vi "Check Tlg.vi"(0 "Data Read In":T1[](array[typedef]) {"FlexRay"."cycle count" max=63 step=1; "payload" format="%x"; "identifier / slot" format="%x"}, 7 "Tlg Data Array":T2 {"CAN frame In"."FlexRay"."cycle count" max=63 step=1; "CAN frame In"."payload" format="%x"; "CAN frame In"."identifier / slot" format="%x"; "FlexRay Channel" items=["A", "B", "A+B"]}, 11 "Error In":errorcluster {"code" format="%.0x"}) -> (4 "Data Read Out":T1[](array[typedef]) {"FlexRay"."cycle count" max=63 step=1; "payload" format="%x"; "identifier / slot" format="%x"}, 8 "Tlg Data Array out":T2 {"CAN frame In"."FlexRay"."cycle count" max=63 step=1; "CAN frame In"."payload" format="%x"; "CAN frame In"."identifier / slot" format="%x"; "FlexRay Channel" items=["A", "B", "A+B"]}, 15 "Error out":errorcluster {"code" format="%.0x"})   [LabVIEW 2014, in "CAN Bus Monitor Engine.lvlib"]
uses:
  CAN Bus Monitor Engine.lvlib
  Controls/Analyze Array.ctl
  Controls/FlexRay Channel.ctl
  Controls/XNET BM Frame.ctl
panel:
  in  "ActualEntry":u32
  in  "EntryFound":bool
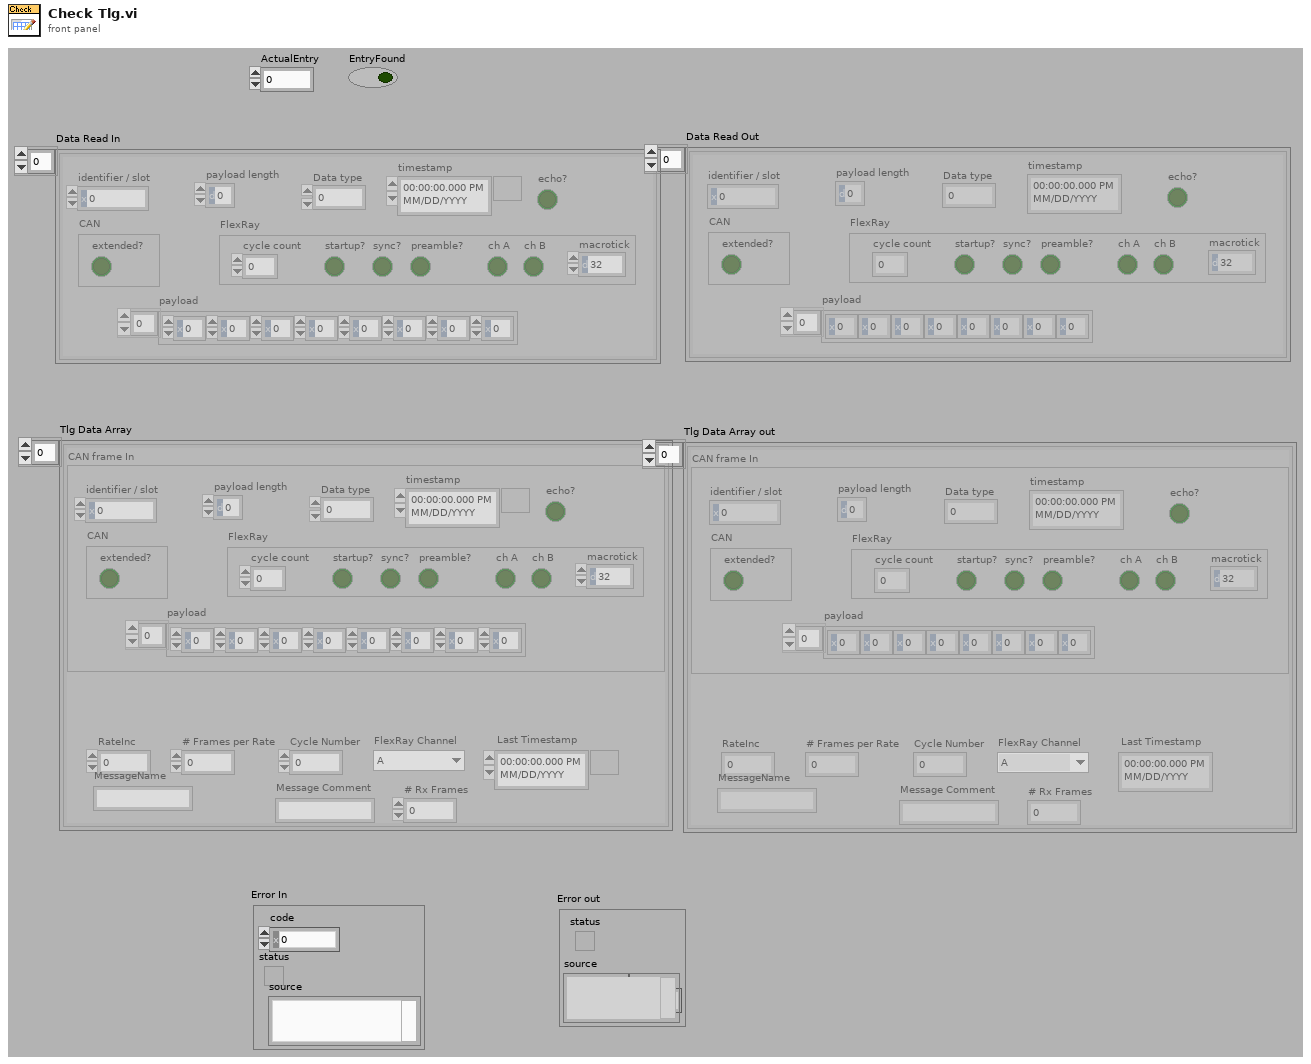
[diagram p1: front panel]
types:
  T1 = typedef "CAN Bus Monitor Engine.lvlib/XNET BM Frame.ctl" = cluster{"timestamp":timestamp, "payload":u8[], "identifier / slot":u32, "Data type":u8, "payload length":u8, "CAN":cluster{"extended?":bool}, "FlexRay":cluster{"cycle count":u8, "startup?":bool, "sync?":bool, "preamble?":bool, "ch A":bool, "ch B":bool, "macrotick":u16}, "echo?":bool}
  T2 = typedef "CAN Bus Monitor Engine.lvlib/Analyze Array.ctl" = cluster{"# Rx Frames":u32, "Last Timestamp":timestamp, "RateInc":dbl, "# Frames per Rate":u32, "MessageName":string, "Cycle Number":u32, "FlexRay Channel":T3, "Message Comment":string, "CAN frame In":T1}[]
  T3 = typedef "CAN Bus Monitor Engine.lvlib/FlexRay Channel.ctl" = u16
  T4 = cluster{"# Rx Frames":u32, "Last Timestamp":timestamp, "RateInc":dbl, "# Frames per Rate":u32, "MessageName":string, "Cycle Number":u32, "FlexRay Channel":T3, "Message Comment":string, "CAN frame In":T1}
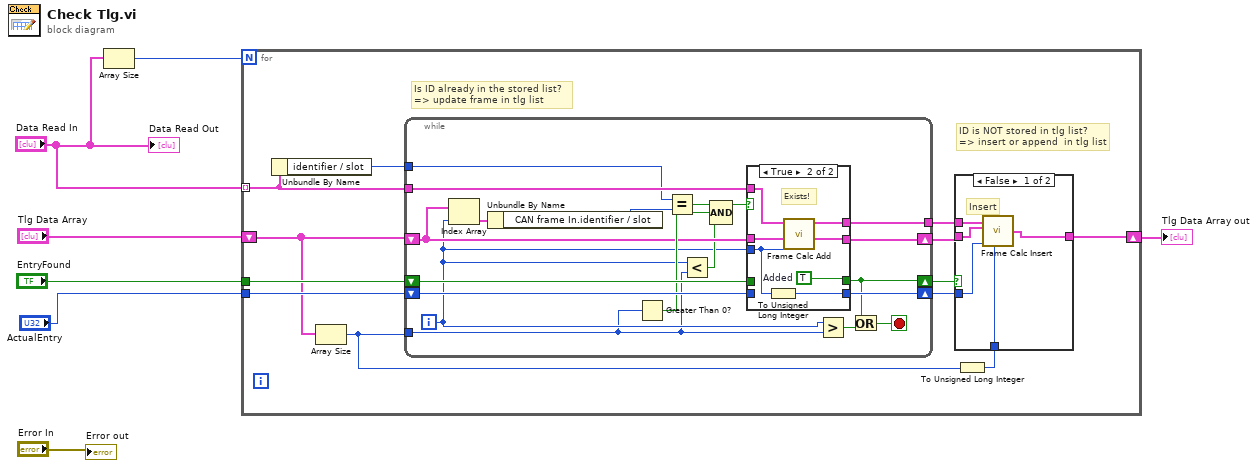
[diagram p0: block diagram]
diagram:
  n1 = Array Size(array="Data Read In") -> (size(s)=w1:i32)
  n2 = for {
    N: w1 -> [_]
    tunnel: "EntryFound" -> [w19]
    tunnel: "Data Read In" -> [w9] mode=indexing
    tunnel: "ActualEntry" -> [w17]
    shift-right: [w18] -> w4
    shift-left: "Tlg Data Array" -> [w11]
    # "ID is NOT stored in tlg list?\n=> insert or append  in tlg list"
    # "Is ID already in the stored list?\n=> update frame in tlg list"
    n3 = Unbundle By Name(w9) -> ("identifier / slot"=w12:u32)
    n4 = Array Size(array=w11) -> (size(s)=w10:i32)
    n5 = while {
      tunnel: w9 -> [w35]
      shift-right: [w40] -> w15
      shift-left: w17 -> [w41]
      shift-right: [w36] -> w14
      shift-left: w19 -> [w44]
      tunnel: w10 -> [w26]
      tunnel: [w34] -> w13
      shift-right: [w39] -> w16
      shift-left: w11 -> [w30]
      tunnel: w12 -> [w31]
      i -> [w27]
      stop <- w38 stop-if-true
      n6 = Index Array(array=w30, index=w27) -> (element=w29:T4)
      n7 = Unbundle By Name(w29) -> ("CAN frame In.identifier / slot"=w42:u32)
      n8 = Greater Than 0?(x=w26) -> (x > 0?=w32:bool)
      n9 = Equal?(x=w31, y=w42) -> (x = y?=w43:bool)
      n10 = Less?(x=w27, y=w26) -> (x < y?=w28:bool)
      n11 = Compound Arithmetic op=AND(w43, w32, w28) -> (w33:bool)
      n12 = case shown="True" w33 {
        tunnel: w44 -> [w46 _]
        tunnel: w41 -> [w48 _]
        tunnel: [w48 w49] -> w40
        tunnel: w27 -> [_ w55]
        tunnel: w30 -> [w47 w54]
        tunnel: [w47 w51] -> w39
        tunnel: [w46 w53] -> w36
        tunnel: w35 -> [w45 w52]
        tunnel: [w45 w50] -> w34
        frame False {
        }
        frame True {
          w53 = TRUE  # Added
          # "Exists!"
          n13 = To Unsigned Long Integer(number=w55) -> (unsigned 32bit integer=w49:u32)
          n14 = call "Frame Calc Add.vi"("Array Position"=w55, "Tlg Data Array In"=w54, "Frame In"=w52) -> ("Tlg Data Array Out"=w51:T2, "Frame Out"=w50:T1)  [unwired: 3 in]
        }
      }
      n15 = Greater?(x=w27, y=w26) -> (0:w37:bool)
      n16 = Or(x=w36, y=w37) -> (x .or. y?=w38:bool)
    }
    n17 = To Unsigned Long Integer(number=w10) -> (unsigned 32bit integer=w8:u32)
    n18 = case shown="False" w14 {
      tunnel: [w24 w25] -> w18
      tunnel: w16 -> [w23 w25]
      tunnel: w15 -> [w22 _]
      tunnel: w8 -> [w21 _]
      tunnel: w13 -> [w20 _]
      frame False {
        # "Insert"
        n19 = call "Frame Calc Insert.vi"("Array Size"=w21, "ActualEntry"=w22, "Tlg Data Array"=w23, "Actual Read frame"=w20) -> ("Tlg Data Array Out"=w24:T2)  [unwired: 2 in]
      }
      frame True {
        # "Frame exists\nand is updated"
      }
    }
  }
  "Tlg Data Array out" <- w4
  "Error out" <- "Error In"
  "Data Read Out" <- "Data Read In"
